vi "Read Key I16.vi"(7 "Section Name":string, 8 "error in":errorcluster, 9 "Default Value":i16, 10 "Key Name":string, 11 "Config File":T1) -> (0 "error out":errorcluster, 1 "Value":i16, 2 "Found?":bool, 3 "Config File":T1)   [LabVIEW 2017]
uses:
  Config Cluster.ctl
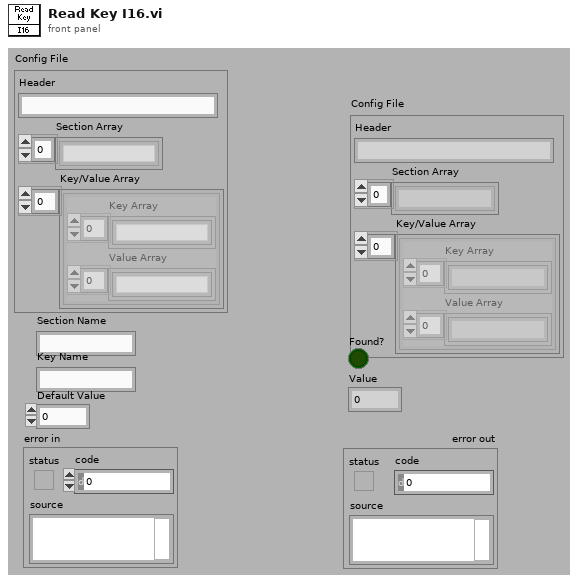
[diagram p1: front panel]
types:
  T1 = typedef "Config Cluster.ctl" = cluster{"Header":string, "Section Array":string[], "Key/Value Array":cluster{"Key Array":string[], "Value Array":string[]}[]}
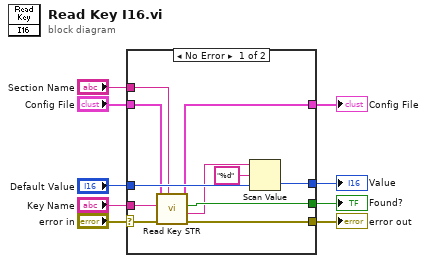
[diagram p0: block diagram]
diagram:
  n1 = case shown="No Error" "error in" {
    selector: "error in" -> [w20 w22]
    tunnel: [w19 w22] -> w8
    tunnel: "Config File" -> [w13 w23]
    tunnel: [w12 w23] -> w6
    tunnel: "Section Name" -> [w11 _]
    tunnel: "Key Name" -> [w10 _]
    tunnel: [w16 w21] -> w3
    tunnel: "Default Value" -> [w17 w21]
    tunnel: [w15 _] -> w1
    frame No Error {
      n2 = call "Read Key STR.vi"("Section Name"=w11, "error in"=w20, "Key Name"=w10, "Config Cluster in"=w13) -> ("error out"=w19:errorcluster, "Value"=w14:string, "Found?"=w15:bool, "Config Cluster out"=w12:T1)  [unwired: 4 in]
      n3 = Scan Value(string=w14, format string="%d", default (0 dbl)=w17) -> (value=w16:i16)  [unwired: 1 out]
    }
    frame Error {
    }
  }
  "error out" <- w8
  "Config File" <- w6
  "Value" <- w3
  "Found?" <- w1
